vi "VIClose.vi"(2 "FPGA Interface Input":refnum<k20>) -> (1 "Error Output":errorcluster)   [LabVIEW 2012]
uses:
  <vilib>/FPGAPlugInAG/Dynamic/niLvFpga_Close_Dynamic.vi
  <vilib>/rvi/interface/nirviCloseFPGA/nirviCloseFPGA.xnode
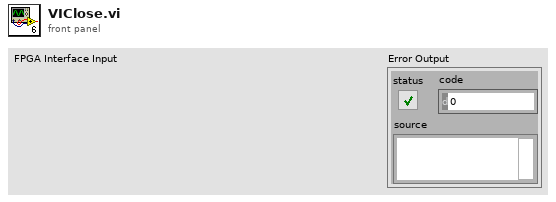
[diagram p1: front panel]
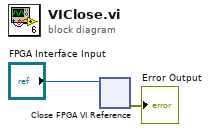
[diagram p0: block diagram]
diagram:
  n1 = xnode "Close FPGA VI Reference"("FPGA VI Reference In"="FPGA Interface Input") -> ("error out"=→"Error Output":errorcluster)  [unwired: 1 in]
